vi "Teleop.vi"(10 "Match Info":T1={"Autonomous Elapsed Seconds"=0.0, "TeleOp Elapsed Seconds"=0.0, "Disabled Elapsed Seconds"=0.0, "Visited Autonomous"=FALSE, "Visited TeleOp"=FALSE, "Visited Disabled"=FALSE, "Autonomous Settings"={"Autonomous Style"=enum."Independent", "VI Refnum"=refnum}}, 11 "Call Context":T2) -> ()   [LabVIEW 2020]
doc: "This VI is called for each TeleOp packet received from the DS where the robot is not disabled. It is often used to read from the joysticks and update I/O or to update setpoints for timed control loops. It should complete and return within 20 milliseconds or it may miss DS packets."
uses:
  <vilib>/Rock Robotics/WPI/DriverStation/WPI_DriverStationDerivedRobotMode.ctl
  <vilib>/Rock Robotics/WPI/DriverStation/WPI_DriverStationMatch Info.ctl
  <vilib>/Rock Robotics/WPI/Solenoid/WPI_SolenoidValue.ctl
  <vilib>/Rock Robotics/WPI/Utilities/WPI_GetSetVariantRefNum.vi
  <vilib>/Rock Robotics/Network Tables/NT Write Boolean Array.vi
  <vilib>/Rock Robotics/Network Tables/NT Write Numeric Array.vi
  <vilib>/Rock Robotics/Network Tables/NT Read Boolean.vi
  <vilib>/Rock Robotics/Network Tables/NT Read Number.vi
  <vilib>/Rock Robotics/WPI/Solenoid/WPI_SolenoidSetEnum.vi
panel:
  out "Sample Slider 0":dbl(slide) scale=0.0..5.0
  out "Sample Boolean 1":bool
  out "Sample Boolean 0":bool
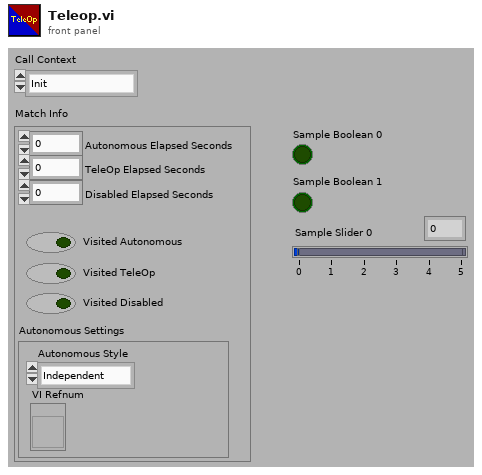
[diagram p1: front panel]
types:
  T1 = typedef "WPI_DriverStationMatch Info.ctl" = cluster{"Autonomous Elapsed Seconds":dbl, "TeleOp Elapsed Seconds":dbl, "Disabled Elapsed Seconds":dbl, "Visited Autonomous":bool, "Visited TeleOp":bool, "Visited Disabled":bool, "Autonomous Settings":cluster{"Autonomous Style":enum16{"Iterative", "Independent"}, "VI Refnum":refnum<vi>}}
  T2 = typedef "WPI_DriverStationDerivedRobotMode.ctl" = enum16{"Init", "Execute", "Stop"}
  T3 = typedef "WPI_SolenoidValue.ctl" = enum16{"Off", "On", "Forward", "Reverse"}
  T4 = typedef "WPI_RobotDriveDevRef.ctl" = cluster{"DevStatus":errorcluster, "Motors[]":T5[], "Square Inputs":bool, "Max Output":dbl}
  T5 = typedef "WPI_MotorControlDeviceRef.ctl" = cluster{"DeviceStatus":errorcluster, "Type":T6, "PWM":cluster{"PWM Channel":T7, "DeadBand":T8}, "CAN":cluster{"Device Number":u8, "SetOutput VI Ref":variant, "GetOutput VI Ref":variant, "Enable VI Ref":variant, "Disable VI Ref":variant, "Data":variant}, "Invert":bool, "DIO PWM":cluster{"PWM \"Enable\" Channel":T7, "DIOChannel":T9, "PWM Rate":dbl}}
  T6 = typedef "WPI_MotorControlType.ctl" = enum16{"PWM", "CAN", "DIO PWM"}
  T7 = typedef "FPGA_DIOPWMChannel.ctl" = enum8{"PWM 0", "PWM 1", "PWM 2", "PWM 3", "PWM 4", "PWM 5", "PWM 6", "PWM 7", "PWM 8", "PWM 9", "PWM MXP 0", "PWM MXP 1", "PWM MXP 2", "PWM MXP 3", "PWM MXP 4", "PWM MXP 5", "PWM MXP 6", "PWM MXP 7", "PWM MXP 8", "PWM MXP 9", "Invalid"}
  T8 = typedef "WPI_PWMDeadband.ctl" = cluster{"Name":string, "maxPositivePwm":i32, "minPositivePwm":i32, "centerPwm":i32, "maxNegativePwm":i32, "minNegativePwm":i32, "angularRange":u16}
  T9 = typedef "FPGA_DIOChannel.ctl" = enum8{"DIO 0", "DIO 1", "DIO 2", "DIO 3", "DIO 4", "DIO 5", "DIO 6", "DIO 7", "DIO 8", "DIO 9", "DIO MXP 0", "DIO MXP 1", "DIO MXP 2", "DIO MXP 3", "DIO MXP 4", "DIO MXP 5", "DIO MXP 6", "DIO MXP 7", "DIO MXP 8", "DIO MXP 9", "DIO MXP 10", "DIO MXP 11", "DIO MXP 12", "DIO MXP 13", "DIO MXP 14", "DIO MXP 15", "SPI Port CS1", "SPI Port CS2", "SPI Port CS3", "SPI Port MISO", "SPI Port MOSI", "Invalid"}
  T10 = typedef "WPI_JoystickDevRef.ctl" = cluster{"Device":T11}
  T11 = typedef "WPI_JoystickDeviceEnum.ctl" = enum16{"USB 0", "USB 1", "USB 2", "USB 3", "USB 4", "USB 5"}
  T12 = typedef "WPI_SolenoidDevRef.ctl" = cluster{"DevStatus":errorcluster, "Pneumatics Control Module":u8, "Forward Solenoid Channel":T13, "Reverse Solenoid Channel":T13}
  T13 = typedef "WPI_SolenoidChannel.ctl" = enum8{"Solenoid 0", "Solenoid 1", "Solenoid 2", "Solenoid 3", "Solenoid 4", "Solenoid 5", "Solenoid 6", "Solenoid 7", "Solenoid 8", "Solenoid 9", "Solenoid 10", "Solenoid 11", "Solenoid 12", "Solenoid 13", "Solenoid 14", "Solenoid 15", "Invalid"}
  T14 = typedef "WPI_ServoDeviceRef.ctl" = cluster{"DeviceStatus":errorcluster, "PWM Channel":T7, "DeadBand":T8}
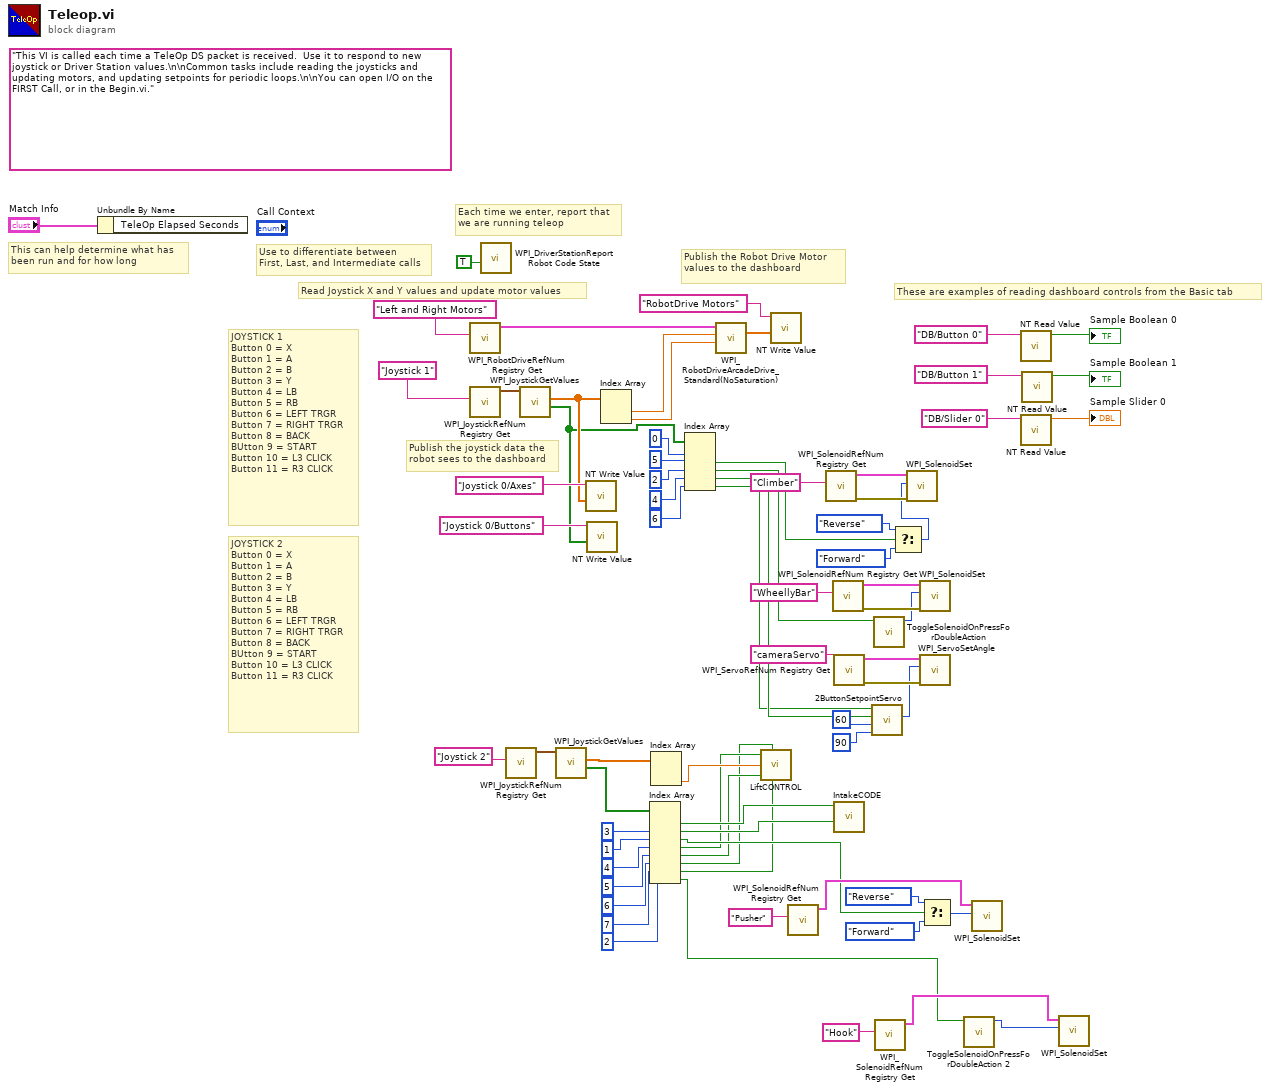
[diagram p0: block diagram]
diagram:
  (unwired) "This VI is called each time a TeleOp DS packet is received.  Use it to respond to new joystick or Driver Station values.\n\nCommon tasks include reading the joysticks and updating motors, and updating setpoints for periodic loops.\n\nYou can open I/O on the FIRST Call, or in the Begin.vi."
  # "JOYSTICK 2\nButton 0 = X\nButton 1 = A\nButton 2 = B\nButton 3 = Y\nButton 4 = LB \nButton 5 = RB\nButton 6 = LEFT TRGR \nButton 7 = RIGHT TRGR \nButton 8 = BACK\nBUtton 9 = START\nButton 10 = L3 CLICK\nButton 11 = R3 CLICK"
  # "JOYSTICK 1\nButton 0 = X\nButton 1 = A\nButton 2 = B\nButton 3 = Y\nButton 4 = LB \nButton 5 = RB\nButton 6 = LEFT TRGR \nButton 7 = RIGHT TRGR \nButton 8 = BACK\nBUtton 9 = START\nButton 10 = L3 CLICK\nButton 11 = R3 CLICK"
  # "These are examples of reading dashboard controls from the Basic tab"
  # "Publish the Robot Drive Motor\nvalues to the dashboard"
  # "Publish the joystick data the\nrobot sees to the dashboard"
  # "Each time we enter, report that\nwe are running teleop"
  # "Use to differentiate between\nFirst, Last, and Intermediate calls"
  # "This can help determine what has\nbeen run and for how long"
  # "Read Joystick X and Y values and update motor values"
  n1 = Unbundle By Name("Match Info") -> ()  [unwired: 1 out]
  n2 = call <vilib>:"WPI_RobotDriveRefNum Registry Get.vi"("refnum name"="Left and Right Motors") -> ("RobotDriveDevRef"=w71:T4)  [unwired: 1 in, 9 out]
  n3 = call <vilib>:"WPI_JoystickRefNum Registry Get.vi"("refnum name"="Joystick 1") -> ("JoystickDevRef"=w68:T10)  [unwired: 1 in, 9 out]
  n4 = call <vilib>:"WPI_DriverStationReport Robot Code State.vi"("TeleOp"=TRUE ("Autonomous")) -> ()  [unwired: 10 in, 1 out]
  n5 = call <vilib>:"WPI_JoystickRefNum Registry Get.vi"("refnum name"="Joystick 2") -> ("JoystickDevRef"=w54:T10)  [unwired: 1 in, 9 out]
  n6 = call <vilib>:"WPI_JoystickGetValues.vi"("JoystickDevRef"=w68) -> ("Buttons"=w51:bool[], "Axes"=w63:dbl[])  [unwired: 6 in, 3 out]
  n7 = call <vilib>:"WPI_JoystickGetValues.vi"("JoystickDevRef"=w54) -> ("Buttons"=w27:bool[], "Axes"=w52:dbl[])  [unwired: 6 in, 3 out]
  n8 = call-poly <vilib>:"NT Write Value.vi"("value"=w63, "name"="Joystick 0/Axes" ("Name")) -> ()  [unwired: 9 in, 1 out]
  n9 = call-poly <vilib>:"NT Write Value.vi"("value"=w51, "name"="Joystick 0/Buttons" ("Name")) -> ()  [unwired: 9 in, 1 out]
  n10 = Index Array(array=w63) -> (element #1=w70:dbl, element #2=w66:dbl)  [unwired: 2 in]
  n11 = Index Array(array=w27, index #2=3 ("index"), index #3=1 ("index"), index #4=4 ("index"), index #5=5 ("index"), index #6=6 ("index"), index #7=7 ("index"), index #8=2 ("index")) -> (element #1=w26:bool, element #2=w18:bool, element #3=w19:bool, element #4=w12:bool, element #5=w11:bool, element #6=w10:bool, element #7=w9:bool, element #8=w2:bool)  [unwired: 1 in]
  n12 = Index Array(array=w52) -> (element #2=w13:dbl)  [unwired: 2 in, 1 out]
  n13 = Index Array(array=w51, index #1=0 ("index"), index #2=5 ("index"), index #3=2 ("index"), index #4=4 ("index"), index #5=6 ("index")) -> (element #2=w43:bool, element #3=w39:bool, element #4=w32:bool, element #5=w31:bool)  [unwired: 1 out]
  n14 = call <vilib>:"WPI_RobotDriveArcadeDrive_Standard(NoSaturation).vi"("Y axis value"=w66, "X axis value"=w70, "RobotDriveDevRef"=w71) -> ("Motor Values"=w56:dbl[])  [unwired: 1 in, 7 out]
  n15 = call "LiftCONTROL.vi"("Left Bumper"=w12, "Left Trigger"=w10, "Manual Control"=w13, "Right Bumper"=w11, "Right Trigger"=w9) -> ()  [unwired: 2 in]
  n16 = call-poly <vilib>:"NT Write Value.vi"("value"=w56, "name"="RobotDrive Motors" ("Name")) -> ()  [unwired: 9 in, 1 out]
  n17 = call <vilib>:"WPI_SolenoidRefNum Registry Get.vi"("refnum name"="Pusher") -> ("SolenoidDevRef"=w22:T12)  [unwired: 9 in, 1 out]
  n18 = call <vilib>:"WPI_SolenoidRefNum Registry Get.vi"("refnum name"="Climber") -> ("error out"=w48:errorcluster, "SolenoidDevRef"=w47:T12)  [unwired: 9 in]
  n19 = call <vilib>:"WPI_SolenoidRefNum Registry Get.vi"("refnum name"="WheellyBar") -> ("error out"=w41:errorcluster, "SolenoidDevRef"=w42:T12)  [unwired: 9 in]
  n20 = call <vilib>:"WPI_ServoRefNum Registry Get.vi"("refnum name"="cameraServo") -> ("error out"=w35:errorcluster, "ServoDeviceRef"=w36:T14)  [unwired: 9 in]
  n21 = call "IntakeCODE.vi"("Intake Button B"=w18, "Intake Button A"=w26) -> ()  [unwired: 9 in, 1 out]
  n22 = call "2ButtonSetpointServo.vi"("Setpoint B"=90 ("Angle"), "Setpoint A"=60 ("Angle"), "Button 1"=w32, "Button 2"=w31) -> ("Value Out"=w28:i32)  [unwired: 7 in]
  n23 = call "ToggleSolenoidOnPressForDoubleAction.vi"("Button"=w39) -> ("Value"=w38:T3)  [unwired: 10 in]
  n24 = call <vilib>:"WPI_SolenoidRefNum Registry Get.vi"("refnum name"="Hook") -> ("SolenoidDevRef"=w5:T12)  [unwired: 9 in, 1 out]
  n25 = Select(t=WPI_SolenoidValue."Reverse" ("Value"), s=w43, f=WPI_SolenoidValue."Forward" ("Value")) -> (s? t:f=w46:T3)
  n26 = call-poly <vilib>:"WPI_SolenoidSet.vi"("error in (no error)"=w48, "Value"=w46, "SolenoidDevRef"=w47) -> ()  [unwired: 7 in, 2 out]
  n27 = call-poly <vilib>:"WPI_SolenoidSet.vi"("error in (no error)"=w41, "Value"=w38, "SolenoidDevRef"=w42) -> ()  [unwired: 7 in, 2 out]
  n28 = call <vilib>:"WPI_ServoSetAngle.vi"("error in (no error)"=w35, "Angle"=w28, "ServoDeviceRef"=w36) -> ()  [unwired: 7 in, 2 out]
  n29 = Select(t=WPI_SolenoidValue."Reverse" ("Value"), s=w19, f=WPI_SolenoidValue."Forward" ("Value")) -> (s? t:f=w23:T3)
  n30 = call "ToggleSolenoidOnPressForDoubleAction 2.vi"("Button"=w2) -> ("Value"=w1:T3)  [unwired: 10 in]
  n31 = call-poly <vilib>:"WPI_SolenoidSet.vi"("Value"=w23, "SolenoidDevRef"=w22) -> ()  [unwired: 8 in, 2 out]
  n32 = call-poly <vilib>:"NT Read Value.vi"("name"="DB/Button 0" ("refnum name")) -> ("value"=→"Sample Boolean 0":bool)  [unwired: 8 in, 2 out]
  n33 = call-poly <vilib>:"NT Read Value.vi"("name"="DB/Slider 0" ("refnum name")) -> ("value"=→"Sample Slider 0":dbl)  [unwired: 8 in, 2 out]
  n34 = call-poly <vilib>:"NT Read Value.vi"("name"="DB/Button 1" ("refnum name")) -> ("value"=→"Sample Boolean 1":bool)  [unwired: 8 in, 2 out]
  n35 = call-poly <vilib>:"WPI_SolenoidSet.vi"("Value"=w1, "SolenoidDevRef"=w5) -> ()  [unwired: 8 in, 2 out]
